vi "Periodic Tasks.vi"(8 "error in":errorcluster) -> ()   [LabVIEW 2017]
doc: "This VI runs in parallel to other robot code. It can contain as many user-defined periodic loops as you need. These can carry out PID or other sorts of timed response."
uses:
  <vilib>/Rock Robotics/Network Tables/NT Read String.vi
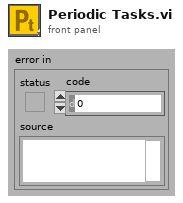
[diagram p1: front panel]
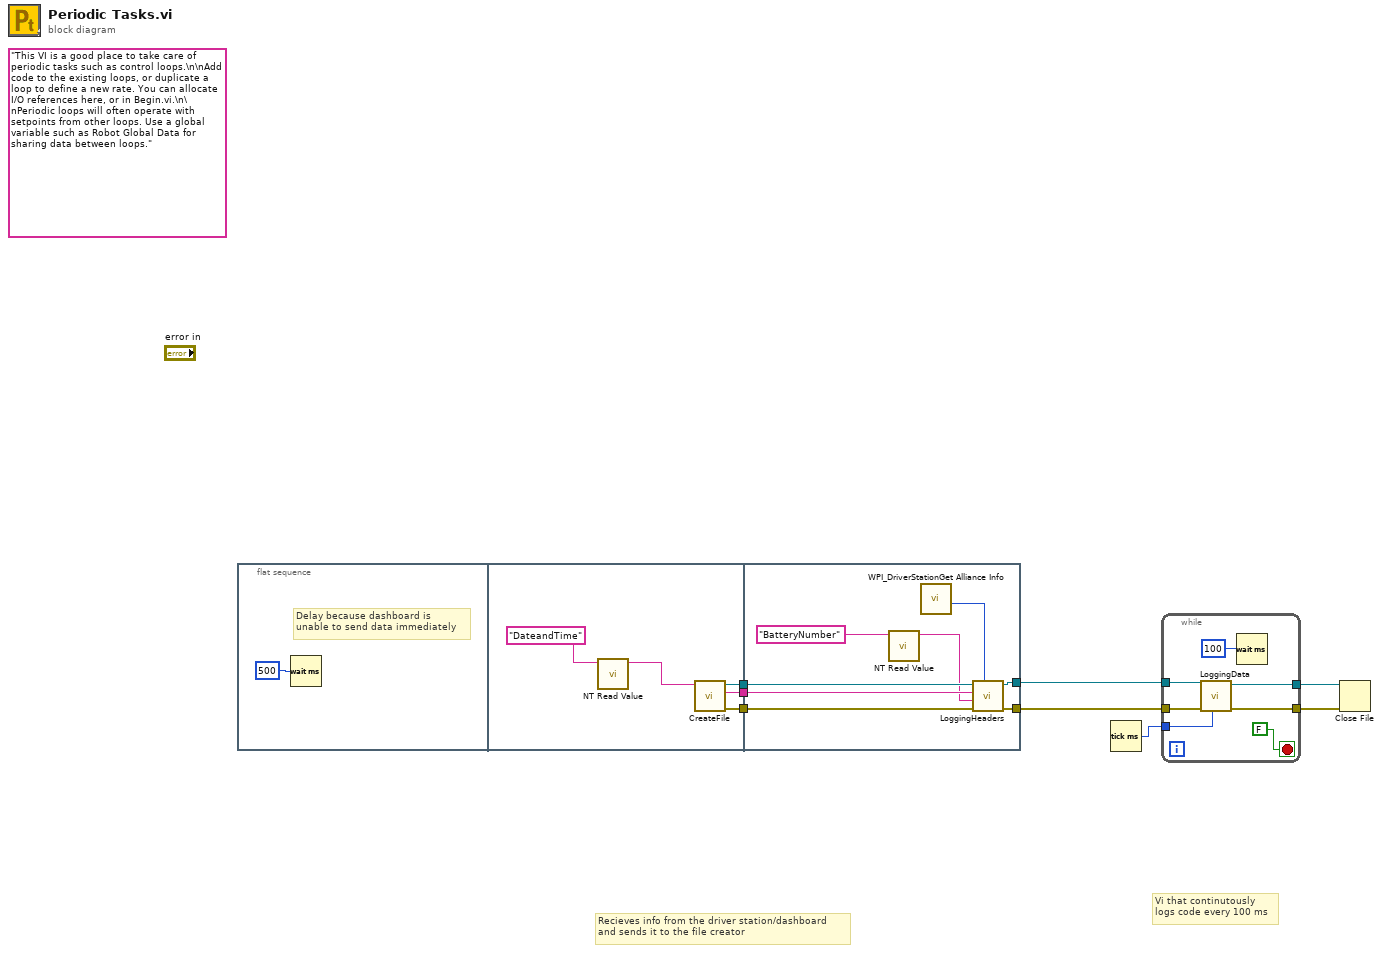
[diagram p0: block diagram]
diagram:
  (unwired) "This VI is a good place to take care of periodic tasks such as control loops.\n\nAdd code to the existing loops, or duplicate a loop to define a new rate. You can allocate I/O references here, or in Begin.vi.\n\nPeriodic loops will often operate with setpoints from other loops. Use a global variable such as Robot Global Data for sharing data between loops."
  # "Vi that continutously\nlogs code every 100 ms"
  # "Recieves info from the driver station/dashboard\nand sends it to the file creator"
  n1 = flat-sequence {
    tunnel: [w13] -> w7
    tunnel: [w14] -> w8
    tunnel: [w12] -> w6
    tunnel: w8 -> [w19]
    tunnel: w7 -> [w20]
    tunnel: [w21] -> w3
    tunnel: [w22] -> w4
    tunnel: w6 -> [w18]
    frame #0 {
      # "Delay because dashboard is \nunable to send data immediately"
      n2 = Wait (ms)(milliseconds to wait=u32 500) -> ()  [unwired: 1 out]
    }
    frame #1 {
      n3 = call-poly <vilib>:"NT Read Value.vi"("Name"="DateandTime") -> ("String"=w11:string)  [unwired: 9 in, 1 out]
      n4 = call "CreateFile.vi"("Date/Time"=w11) -> ("error out"=w12:errorcluster, "Date/Time String"=w14:string, "Refnum Out"=w13:refnum<file>)  [unwired: 8 in]
    }
    frame #2 {
      n5 = call-poly <vilib>:"NT Read Value.vi"("Name"="BatteryNumber") -> ("String"=w17:string)  [unwired: 9 in, 1 out]
      n6 = call <vilib>:"WPI_DriverStationGet Alliance Info.vi"() -> ("Match Number"=w15:u16)  [unwired: 6 in, 5 out]
      n7 = call "LoggingHeaders.vi"("Match Number"=w15, "error in"=w18, "Battery Number"=w17, "Date and Time"=w19, "refnum in"=w20) -> ("error out"=w22:errorcluster, "refnum out"=w21:refnum<file>)  [unwired: 5 in]
    }
  }
  n8 = Tick Count (ms)() -> (millisecond timer value=w5:u32)
  n9 = while {
    tunnel: w5 -> [w29]
    tunnel: [w27] -> w2
    tunnel: [w28] -> w1
    tunnel: w3 -> [w25]
    tunnel: w4 -> [w26]
    stop <- FALSE stop-if-true
    n10 = call "LoggingData.vi"("Start time"=w29, "error in"=w26, "refnum in"=w25) -> ("error out"=w28:errorcluster, "refnum out"=w27:refnum<file>)  [unwired: 7 in]
    n11 = Wait (ms)(milliseconds to wait=u32 100) -> ()  [unwired: 1 out]
  }
  n12 = Close File(refnum=w2, error in=w1) -> ()  [unwired: 2 out]
